vi "String Key Down Filter.vi"(9 "VKey in":T1, 10 "Char in":i16, 11 "Settings UI in":refnum<class "Settings UI.lvclass">) -> (0 "Discard?":bool, 1 "VKey out":T1, 2 "Char out":i16, 3 "Settings UI out":refnum<class "Settings UI.lvclass">)   [LabVIEW 2020, in "Output Sequencer.lvlib" / "Settings UI.lvclass"]
uses:
  Settings UI.lvclass
  <vilib>/event_ctls.llb/eventvkey.ctl
  Settings UI.lvclass/Settings UI.ctl
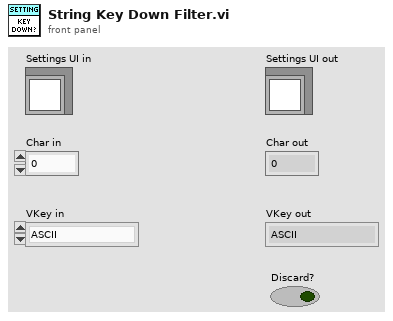
[diagram p1: front panel]
types:
  T1 = typedef "eventvkey.ctl" = enum16{"ASCII", "Enter", "Return", "Shift", "Ctrl", "Alt", "Cmd", "Opt", "Caps", "NumLock", "Clear", "Break", "Up", "Down", "Left", "Right", "Insert", "Delete", "Home", "End", "PageUp", "PageDown", "Escape", "Help", "Pause", "ScrollLock", "F1", "F2", "F3", "F4", "F5", "F6", "F7", "F8", "F9", "F10", "F11", "F12", "F13", "F14", "F15", "F16", "F17", "F18", "F19", "F20", "F21", "F22", "F23", "F24", "Play", "VolumeUp", "VolumeDown", "Mute", "Two Byte Char"}
  T2 = typedef "Output Sequencer.lvlib/Settings UI.lvclass/Autocomplete State.ctl" = cluster{"Variables":string[], "Active?":bool, "Search Offset":i32, "Matches":i32[], "Match Index":i32}
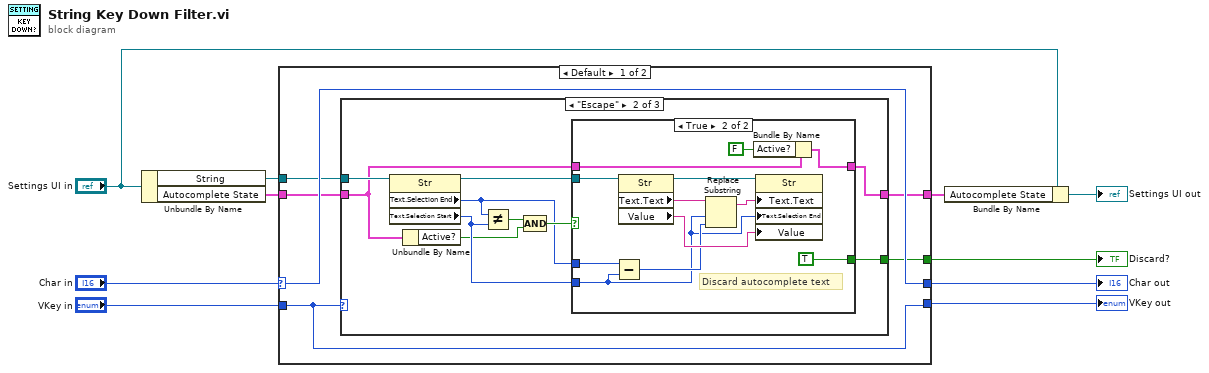
[diagram p0: block diagram]
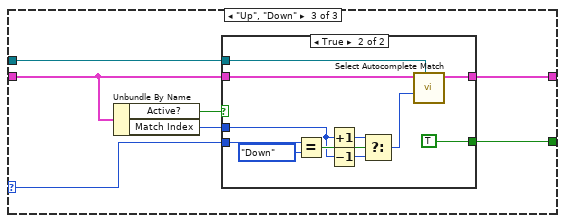
[diagram p4: hidden frame]
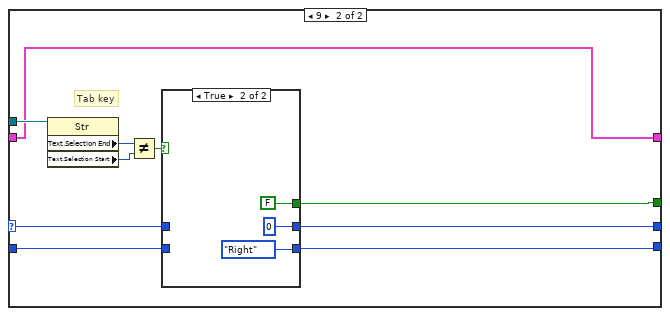
[diagram p6: hidden frame]
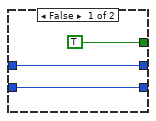
[diagram p7: hidden frame]
diagram:
  n1 = Unbundle By Name("Settings UI in") -> ("String"=w7:refnum<vi>, "Autocomplete State"=w8:T2)
  n2 = case shown="Default" "Char in" {
    selector: "Char in" -> [w16 w66]
    tunnel: w7 -> [w15 w69]
    tunnel: [w13 w64] -> w2
    tunnel: [w16 w67] -> w4
    tunnel: [w14 w65] -> w5
    tunnel: "VKey in" -> [w14 w68]
    tunnel: w8 -> [w12 w60]
    tunnel: [w11 w60] -> w9
    frame Default {
      n3 = case shown="\"Escape\"" w14 {
        selector: w14 -> [_ _ w44]
        tunnel: w15 -> [_ w27 w43]
        tunnel: [_ w22 w47] -> w13
        tunnel: w12 -> [w17 w19 w42]
        tunnel: [w17 w18 w41] -> w11
        frame Default {
        }
        frame "Escape" {
          n4 = property class="Str"(reference=w27) -> (reference out=w26:refnum<vi>, "Text.Selection End"=w20:u32, "Text.Selection Start"=w25:u32)  [unwired: 1 in, 1 out]
          n5 = Unbundle By Name(w19) -> ("Active?"=w21:bool)
          n6 = Not Equal?(x=w20, y=w25) -> (x != y?=w24:bool)
          n7 = Compound Arithmetic op=AND(w24, w21) -> (w23:bool)
          n8 = case shown="True" w23 {
            tunnel: w26 -> [_ w40]
            tunnel: w25 -> [_ w30]
            tunnel: [_ TRUE ("AutoComplete active")] -> w22
            tunnel: w19 -> [w28 w36]
            tunnel: w20 -> [_ w32]
            tunnel: [w28 w29] -> w18
            frame False {
            }
            frame True {
              # "Discard autocomplete text"
              n9 = Subtract(x=w32, y=w30) -> (x-y=w31:u32)
              n10 = property class="Str"(reference=w40) -> (reference out=w38:refnum<vi>, "Text.Text"=w34:string, "Value"=w37:string)  [unwired: 1 in, 1 out]
              n11 = Replace Substring(2:w31, 3:w30, 5:w34) -> (1:w33:string)  [unwired: 1 in, 1 out]
              n12 = Bundle By Name(cluster=w36, "Active?"=FALSE ("AutoComplete active")) -> (w29:T2)
              n13 = property class="Str"(reference=w38, "Text.Text"=w33, "Text.Selection End"=w30, "Value"=w37) -> ()  [unwired: 1 in, 2 out]
            }
          }
        }
        frame "Up", "Down" {
          n14 = Unbundle By Name(w42) -> ("Active?"=w46:bool, "Match Index"=w45:i32)
          n15 = case shown="True" w46 {
            tunnel: [_ TRUE] -> w47
            tunnel: w45 -> [_ w54]
            tunnel: w44 -> [_ w53]
            tunnel: w42 -> [w48 w51]
            tunnel: w43 -> [_ w50]
            tunnel: [w48 w49] -> w41
            frame False {
            }
            frame True {
              n16 = Equal?(x=w53, y=eventvkey."Down") -> (x = y?=w57:bool)
              n17 = Increment(x=w54) -> (x+1=w56:i32)
              n18 = Decrement(x=w54) -> (x-1=w55:i32)
              n19 = Select(t=w56, s=w57, f=w55) -> (s? t:f=w52:i32)
              n20 = call "Select Autocomplete Match.vi"("String in"=w50, "Match Index"=w52, "Autocomplete State in"=w51) -> ("Autocomplete State out"=w49:T2)  [unwired: 8 in]
            }
          }
        }
      }
    }
    frame 9 {
      # "Tab key"
      n21 = property class="Str"(reference=w69) -> ("Text.Selection End"=w61:u32, "Text.Selection Start"=w63:u32)  [unwired: 1 in, 2 out]
      n22 = Not Equal?(x=w61, y=w63) -> (x != y?=w62:bool)
      n23 = case shown="True" w62 {
        tunnel: w68 -> [w71 _]
        tunnel: [w72 i16 0 ("Char")] -> w67
        tunnel: w66 -> [w72 _]
        tunnel: [w71 eventvkey."Right" ("VKey")] -> w65
        tunnel: [TRUE FALSE] -> w64
        frame False {
        }
        frame True {
        }
      }
    }
  }
  "VKey out" <- w5
  "Char out" <- w4
  "Discard?" <- w2
  n24 = Bundle By Name(cluster="Settings UI in", "Autocomplete State"=w9) -> (→"Settings UI out":refnum<class "Settings UI.lvclass">)
